vi "SetTrigSource.vi"(8 "TrigSource":u8, 11 "error in":errorcluster caption="错误输入") -> (3 "error out":errorcluster caption="错误输出")   [LabVIEW 2016]
uses:
  PLC-Lab/lib/gusb.dll
panel:
  # "0: soft trig\n1~8: digital in 0 ~ digital in 7"
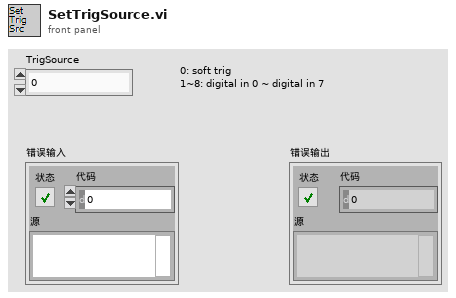
[diagram p1: front panel]
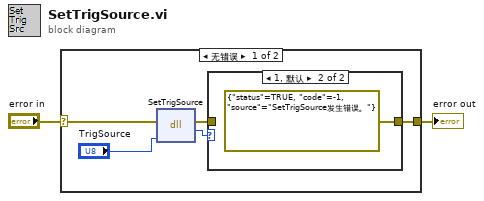
[diagram p0: block diagram]
diagram:
  n1 = case shown="无错误" "error in" {
    selector: "error in" -> [w7 w10]
    tunnel: [w5 w10] -> w1
    frame No Error {
      n2 = dll-call lib="E:/Camproject/2018/2018.1Labview/PLC-Lab/lib/gusb.dll" fn="SetTrigSource"(error in=w7, "TrigSource"="TrigSource") -> (error out=w4:errorcluster, "Status"=w6:i32)  [unwired: 3 in, 1 out]
      n3 = case shown="1, 默认" w6 {
        tunnel: w4 -> [w8 _]
        tunnel: [w8 errorcluster {"status"=TRUE, "code"=-1, "source"="SetTrigSource发生错误。"} ("错误常量")] -> w5
        frame 0 {
        }
        frame 1, Default {
        }
      }
    }
    frame Error {
    }
  }
  "error out" <- w1
